vi "r1.vi"   [LabVIEW 2019]
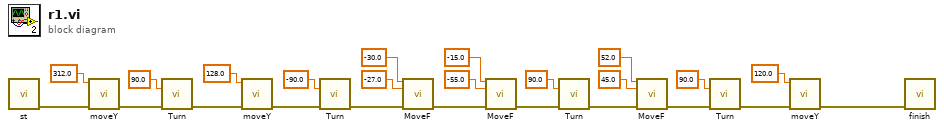
[diagram p0: block diagram]
diagram:
  n1 = call "st.vi"() -> ("Error/Flow Out"=w24:errorcluster)  [unwired: 11 in]
  n2 = call "moveY.vi"("error in (no error)"=w24, "Y"=312.0) -> ("error out"=w22:errorcluster)  [unwired: 9 in]
  n3 = call "Turn.vi"("¨¤«×"=90.0, "error in (no error)"=w22) -> ("error out"=w19:errorcluster)  [unwired: 13 in]
  n4 = call "moveY.vi"("error in (no error)"=w19, "Y"=128.0) -> ("error out"=w17:errorcluster)  [unwired: 9 in]
  n5 = call "Turn.vi"("¨¤«×"=-90.0, "error in (no error)"=w17) -> ("error out"=w16:errorcluster)  [unwired: 13 in]
  n6 = call "MoveF.vi"("X"=-30.0, "Y"=-27.0, "error in (no error)"=w16) -> ("error out"=w11:errorcluster)  [unwired: 12 in]
  n7 = call "MoveF.vi"("X"=-15.0, "Y"=-55.0, "error in (no error)"=w11) -> ("error out"=w9:errorcluster)  [unwired: 12 in]
  n8 = call "Turn.vi"("¨¤«×"=90.0, "error in (no error)"=w9) -> ("error out"=w6:errorcluster)  [unwired: 13 in]
  n9 = call "MoveF.vi"("X"=52.0, "Y"=45.0, "error in (no error)"=w6) -> ("error out"=w4:errorcluster)  [unwired: 12 in]
  n10 = call "Turn.vi"("¨¤«×"=90.0, "error in (no error)"=w4) -> ("error out"=w2:errorcluster)  [unwired: 13 in]
  n11 = call "moveY.vi"("error in (no error)"=w2, "Y"=120.0) -> ("error out"=w1:errorcluster)  [unwired: 9 in]
  n12 = call "finish.vi"("Error/Flow In"=w1) -> ()  [unwired: 11 in]
